vi "Channel(9600).vi"(7 "Выборка\nс передатчика":cdb format="%#.6g") -> (8 "Выборка \nс канала":cdb)   [LabVIEW 2013]
uses:
  <vilib>/ptbypt/NI_PtbyPt.lvlib
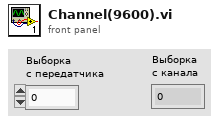
[diagram p1: front panel]
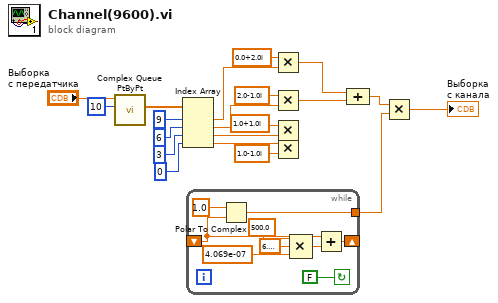
[diagram p0: block diagram]
diagram:
  n1 = call <vilib>:"Complex Queue PtByPt.vi"("sample length"=10, "input data point"="Выборка\nс передатчика") -> ("Current Queue"=w18:cdb[])  [unwired: 5 in, 4 out]
  n2 = Index Array(array=w18, index #1=9 ("index"), index #2=6 ("index"), index #3=3 ("index"), index #4=0 ("index")) -> (element #1=w13:cdb, element #2=w12:cdb, element #3=w11:cdb, element #4=w10:cdb)
  n3 = while {
    shift-right: [w24] -> _
    shift-left: _ -> [w23]
    tunnel: [w21] -> w3
    stop <- FALSE continue-if-true
    n4 = Polar To Complex(1:w23, 2:1.0 ("r")) -> (0:w21:cdb)
    n5 = Compound Arithmetic op=MULTIPLY(500.0, 6.283185307179586, 4.069e-07 ("value")) -> (w25:dbl)
    n6 = Add(x=w23, y=w25) -> (x+y=w24:dbl)
  }
  n7 = Multiply(x=cdb 0.0+2.0i, y=w13) -> (x*y=w5:cdb)
  n8 = Multiply(x=cdb 2.0-1.0i, y=w12) -> (x*y=w1:cdb)
  n9 = Multiply(x=cdb 1.0+1.0i, y=w11) -> ()  [unwired: 1 out]
  n10 = Multiply(x=w10, y=cdb 1.0-1.0i) -> ()  [unwired: 1 out]
  n11 = Compound Arithmetic op=ADD(w5, w1) -> (w4:cdb)
  n12 = Multiply(x=w4, y=w3) -> (x*y=→"Выборка \nс канала":cdb)
